vi "Get ECUMC Value.vi"(8 "Error In":errorcluster, 11 "Link":T1) -> (0 "Error Out":errorcluster, 2 "Changed?":bool, 3 "Value":dbl)   [LabVIEW 2011]
uses:
  Controls/ECUMC Item.ctl
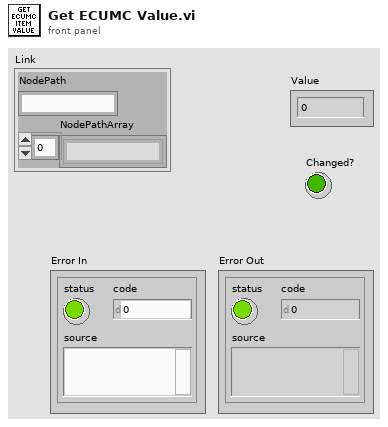
[diagram p1: front panel]
types:
  T1 = typedef "ECUMC Item.ctl" = cluster{"NodePath":string, "NodePathArray":string[]}
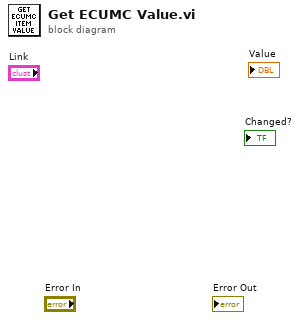
[diagram p0: block diagram]
diagram:
